vi "Tracking with Motor.vi"(6 "Speed Control":dbl, 8 "Right Limit":bool, 9 "Left Limit":bool, 10 "Tolerance":dbl, 11 "Actual Position (x)":dbl) -> ()   [LabVIEW 2011]
panel:
  out "Limit \nReached!":bool
  out "Centered Postion":dbl
  out "Fire!":bool
  out "Right Boundary":dbl
  out "Left Boundary":dbl
  # "Center (x = 0)"
  # "Left Bound = Target - Tolerance"
  # "Backboard"
  # "Right Bound = Target + Tolerance"
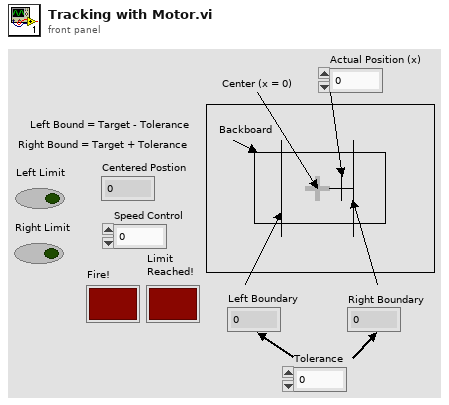
[diagram p1: front panel]
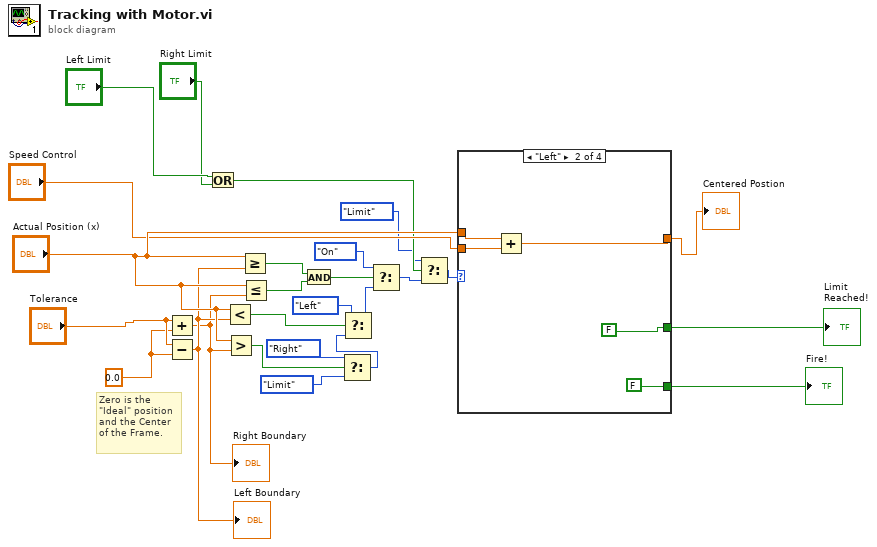
[diagram p0: block diagram]
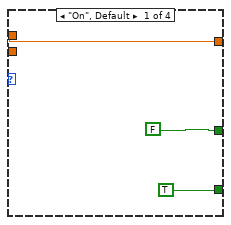
[diagram p2: hidden frame]
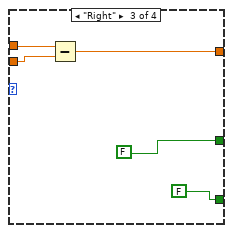
[diagram p3: hidden frame]
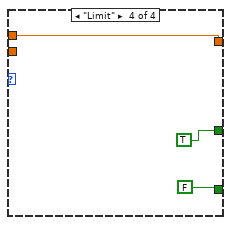
[diagram p4: hidden frame]
diagram:
  w19 = 0.0
  # "Zero is the \n\"Ideal\" position\nand the Center \nof the Frame."
  n1 = Add(x="Tolerance", y=w19) -> (x+y=w10:dbl)
  "Right Boundary" <- w10
  n2 = Subtract(x="Tolerance", y=w19) -> (x-y=w14:dbl)
  "Left Boundary" <- w14
  n3 = Or(x="Left Limit", y="Right Limit") -> (x .or. y?=w3:bool)
  n4 = Less?(x="Actual Position (x)", y=w14) -> (x < y?=w12:bool)
  n5 = Greater?(x="Actual Position (x)", y=w10) -> (0:w7:bool)
  n6 = Greater Or Equal?(x="Actual Position (x)", y=w14) -> (x >= y?=w18:bool)
  n7 = Less Or Equal?(x="Actual Position (x)", y=w10) -> (x <= y?=w17:bool)
  n8 = And(x=w18, y=w17) -> (x .and. y?=w16:bool)
  n9 = Select(t=enum16{"On", "Left", "Right", "Limit"}."Right", s=w7, f=enum16{"On", "Left", "Right", "Limit"}."Limit") -> (s? t:f=w9:enum16{"On", "Left", "Right", "Limit"})
  n10 = Select(t=enum16{"On", "Left", "Right", "Limit"}."Left", s=w12, f=w9) -> (s? t:f=w13:enum16{"On", "Left", "Right", "Limit"})
  n11 = Select(t=enum16{"On", "Left", "Right", "Limit"}."On", s=w16, f=w13) -> (s? t:f=w5:enum16{"On", "Left", "Right", "Limit"})
  n12 = Select(t=enum16{"On", "Left", "Right", "Limit"}."Limit", s=w3, f=w5) -> (s? t:f=w4:enum16{"On", "Left", "Right", "Limit"})
  n13 = case shown="\"Left\"" w4 {
    tunnel: [w29 w33 w39 w40] -> w1
    tunnel: "Actual Position (x)" -> [w29 w34 w38 w40]
    tunnel: [TRUE FALSE ("Fire!") FALSE FALSE] -> w24
    tunnel: "Speed Control" -> [_ w31 w36 _]
    tunnel: [FALSE ("Fire!") FALSE ("Fire!") FALSE ("Fire!") TRUE] -> w20
    frame "On", Default {
    }
    frame "Left" {
      n14 = Add(x=w34, y=w31) -> (x+y=w33:dbl)
    }
    frame "Right" {
      n15 = Subtract(x=w38, y=w36) -> (x-y=w39:dbl)
    }
    frame "Limit" {
    }
  }
  "Fire!" <- w24
  "Limit \nReached!" <- w20
  "Centered Postion" <- w1
